vi "Traverse_to_Traverse_Collision.vi"(5 "Current Position":dbl[](array[numeric])=[0.0, 100.0, 40.0] format="%.2f", 7 "Traverse Name":string, 8 "Model  Roll        Pitch       Yaw (deg)":dbl[](array[numeric]) format="%#.2f", 9 "Work in Tunnel Coordinates":T1, 10 "Simulate/Run":T2=enum."Run VI", 11 "New Position":dbl[](array[numeric])=[0.0, 100.0, 40.0] format="%.2f") -> (1 "Error String":string)   [LabVIEW 2012]
uses:
  Controls/User_Specific_mode.ctl
  Controls/Tunnel_Coordinates.ctl
  Route mapping/Exclude_cluster.ctl
  Route mapping/Box_size.ctl
  Route mapping/Exclusion_type.ctl
  Controls/Global_mode.ctl
  Route mapping/Pict_Plot_Axis.ctl
  Route mapping/Axis.ctl
  Globals/Preference_global.vi
  Globals/Trav_pos_global.vi
panel:
  out "Plan View":picture
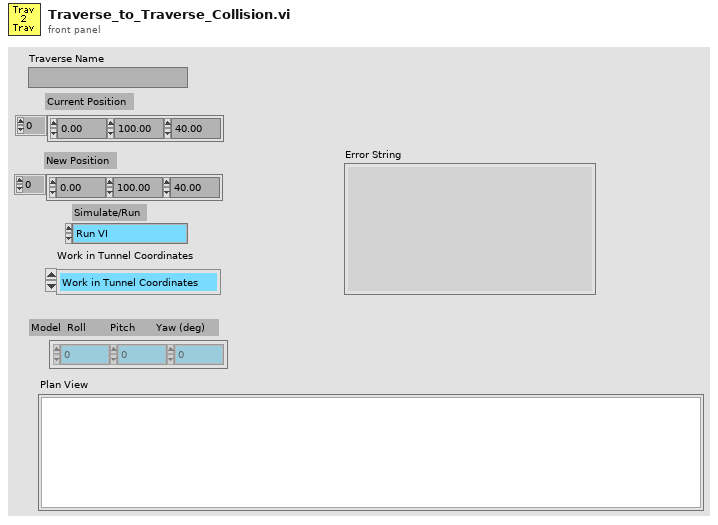
[diagram p1: front panel]
types:
  T1 = typedef "Tunnel_Coordinates.ctl" = enum16{"Work in Tunnel Coordinates", "Work in Model Coordinates"}
  T2 = typedef "User_Specific_mode.ctl" = enum16{"Check VI only", "Run VI"}
  T3 = typedef "Exclude_cluster.ctl" = cluster{"Sizes":T4, "Name":string, "Exclude Type":T5}
  T4 = typedef "Box_size.ctl" = cluster{"Max":dbl, "Min":dbl}[]
  T5 = typedef "Exclusion_type.ctl" = enum16{"Exclude completely", "Allow only vertical moves"}
  T6 = typedef "Global_mode.ctl" = enum16{"Read Global", "Load Global From File", "Write Global to File"}
  T7 = typedef "Pict_Plot_Axis.ctl" = cluster{"Width":T8, "Height":T8}
  T8 = typedef "Axis.ctl" = enum16{"X Axis", "X Axis -ve", "Y Axis", "Y Axis -ve", "Z Axis", "Z Axis -ve"}
  T9 = typedef "Update_scan_value.ctl" = cluster{"Channel Name":string, "New Value":dbl}
  T10 = enum16{"To Traverse Coordinates", "To User Coordinates"}
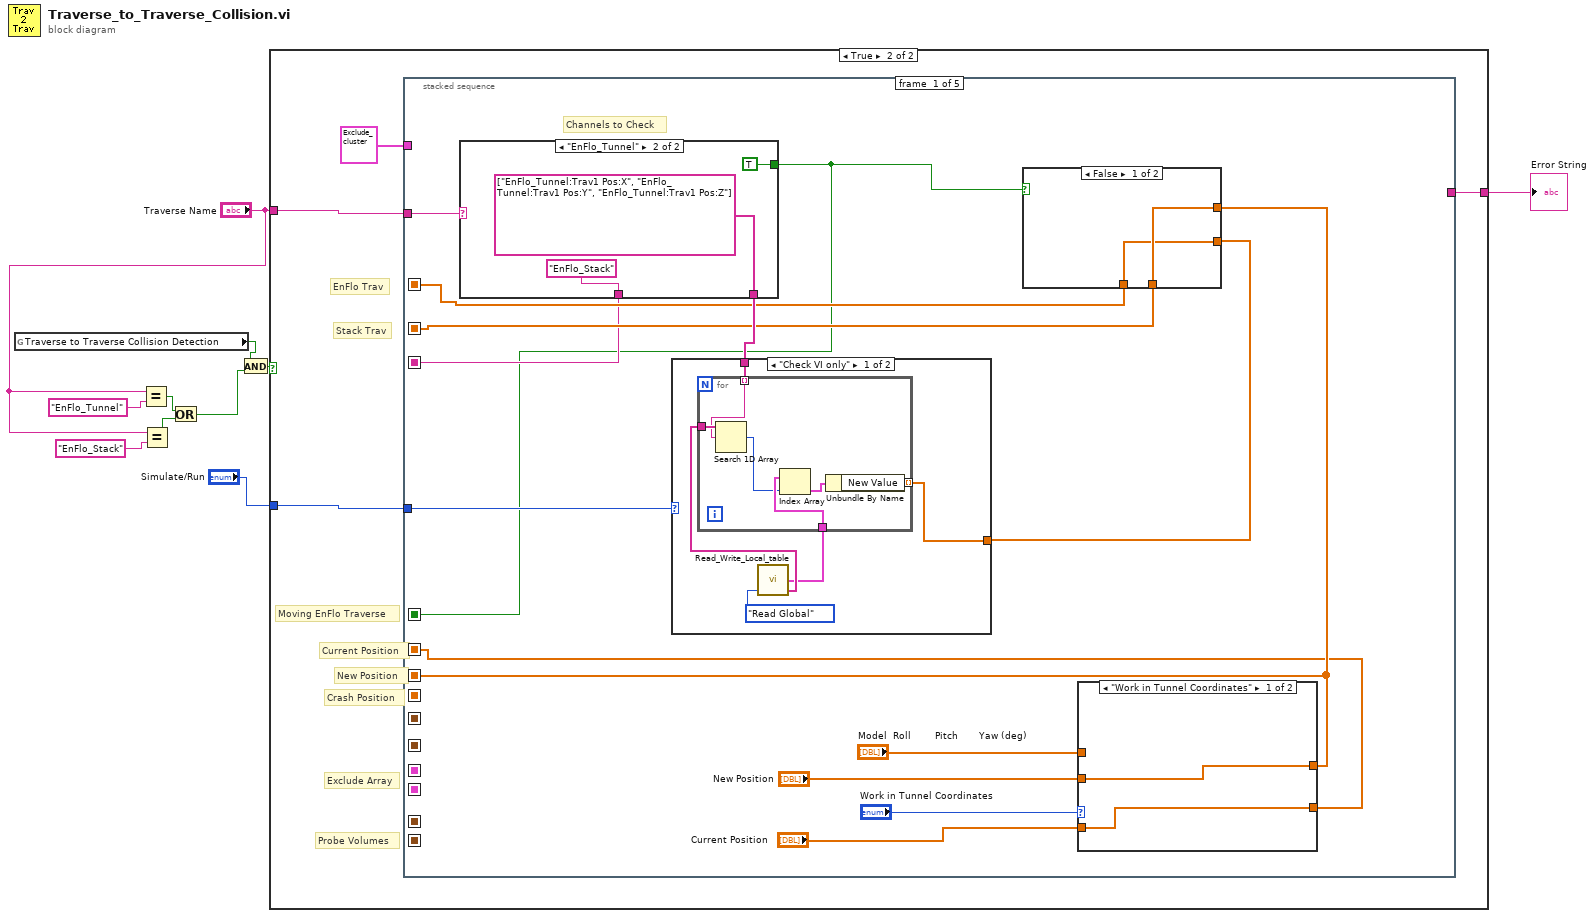
[diagram p0: block diagram]
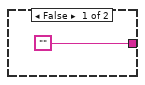
[diagram p2: hidden frame]
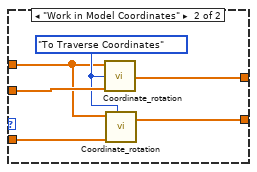
[diagram p4: hidden frame]
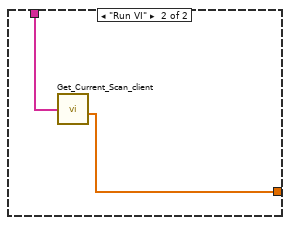
[diagram p5: hidden frame]
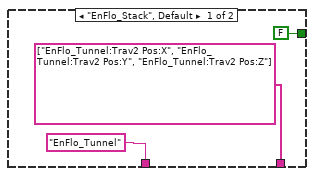
[diagram p6: hidden frame]
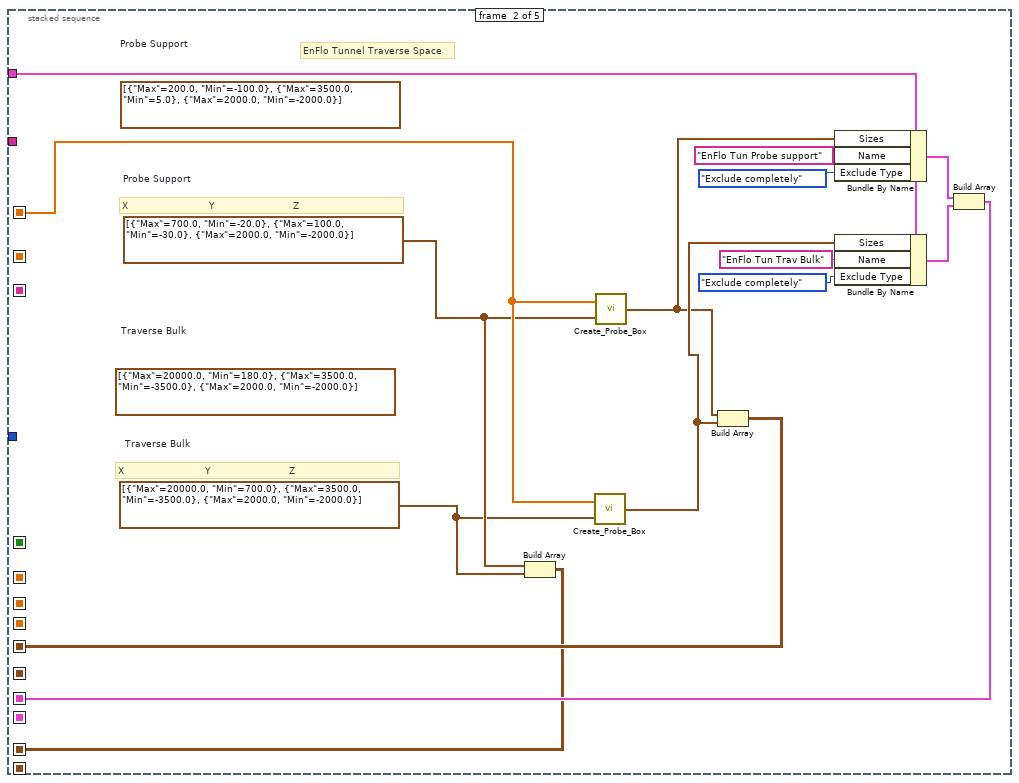
[diagram p7: hidden frame]
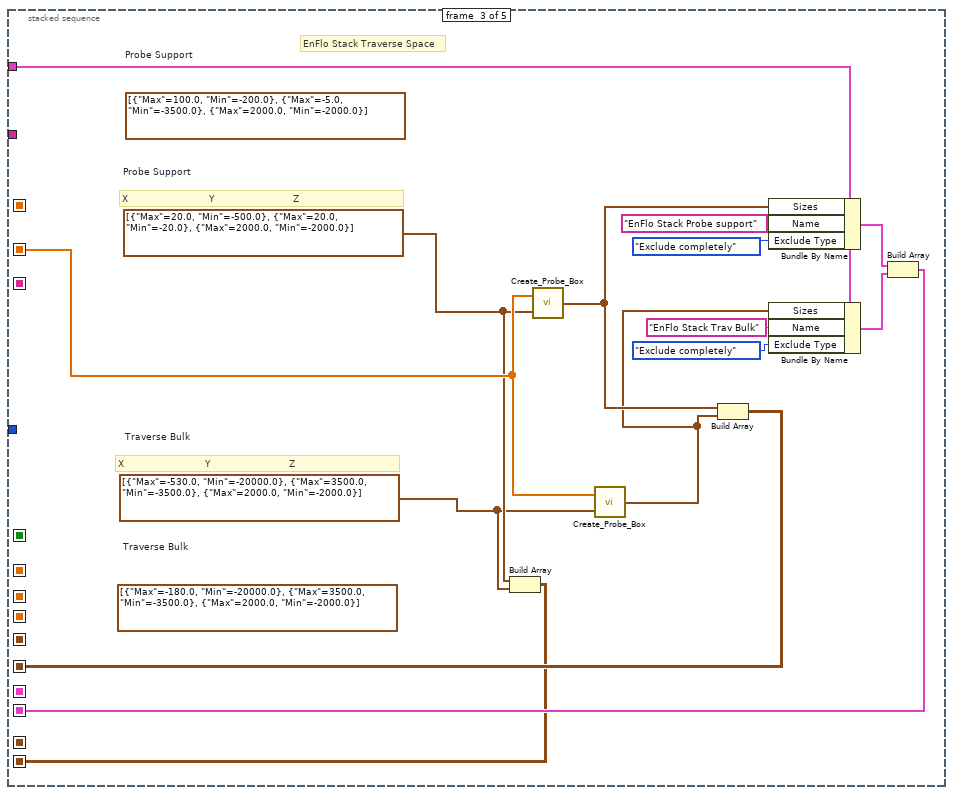
[diagram p8: hidden frame]
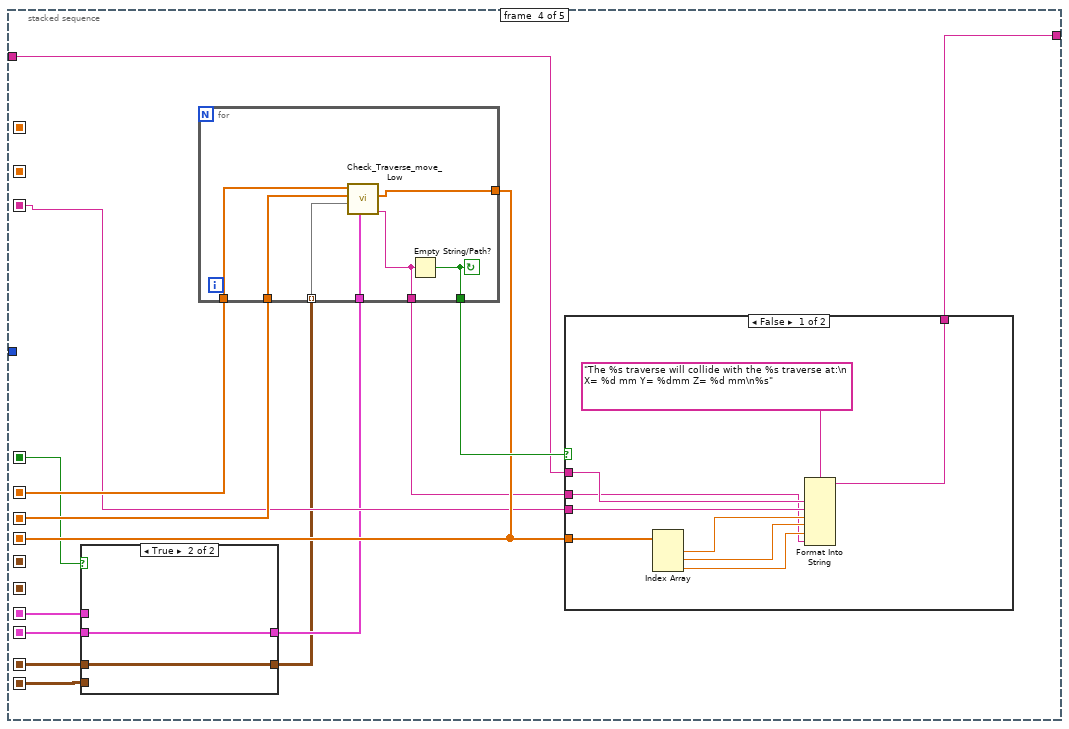
[diagram p9: hidden frame]
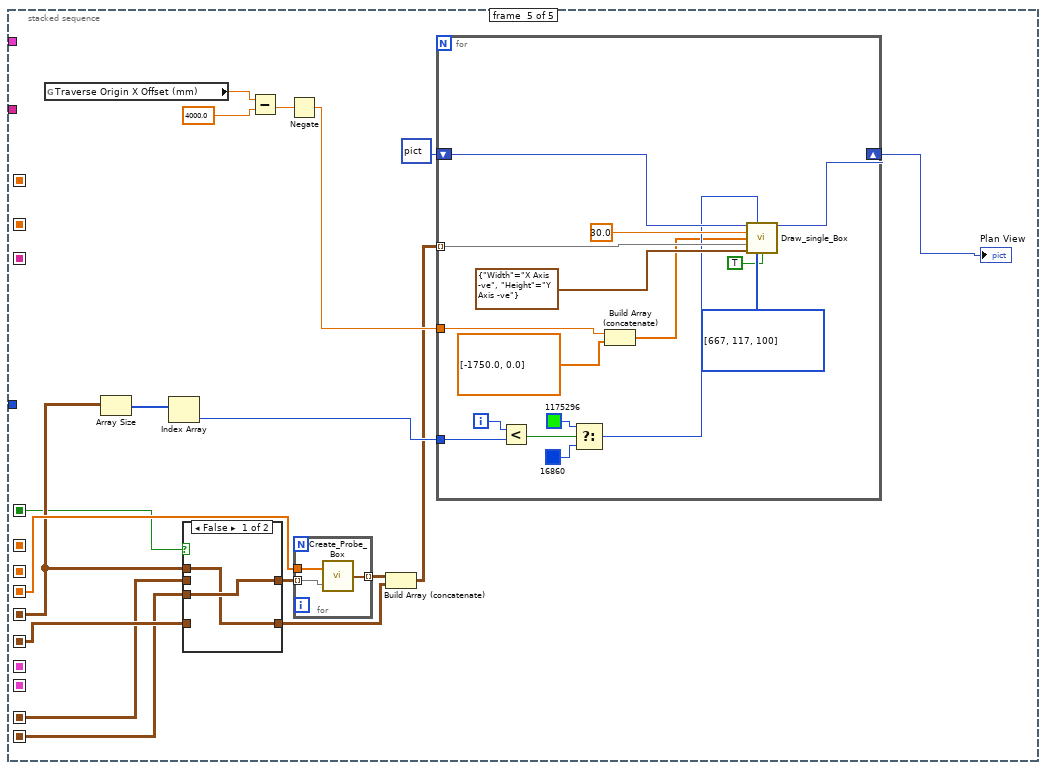
[diagram p12: hidden frame]
diagram:
  n1 = global read "Preference_global.vi" "Traverse to Traverse Collision Detection"() -> (w6:bool)
  n2 = Equal?(x="Traverse Name", y="EnFlo_Tunnel" ("Rig Setup")) -> (x = y?=w3:bool)
  n3 = Equal?(x="Traverse Name", y="EnFlo_Stack" ("Rig Setup")) -> (x = y?=w2:bool)
  n4 = Or(x=w3, y=w2) -> (x .or. y?=w1:bool)
  n5 = And(x=w6, y=w1) -> (x .and. y?=w7:bool)
  n6 = case shown="True" w7 {
    tunnel: "Traverse Name" -> [_ w15]
    tunnel: "Simulate/Run" -> [_ w14]
    tunnel: ["" w13] -> w8
    frame False {
    }
    frame True {
      # "Moving EnFlo Traverse"
      # "Exclude Array"
      # "Probe Volumes"
      # "Crash Position"
      # "Current Position"
      # "New Position"
      # "Stack Trav"
      # "EnFlo Trav"
      n7 = stacked-sequence {
        seq-local: [w23 _ _ _ _] -> [_ w75 _ _ _]
        seq-local: [w22 _ _ _ _] -> [_ _ w89 _ _]
        seq-local: [_ w74 _ _ _] -> [_ _ _ _ w128]
        seq-local: [_ _ w90 _ _] -> [_ _ _ _ w135]
        seq-local: [w20 _ _ _ _] -> [_ _ _ w100 _]
        seq-local: [w19 _ _ _ _] -> [_ _ _ w105 _]
        seq-local: [_ _ w80 _ _] -> [_ _ _ w97 _]
        seq-local: [_ w64 _ _ _] -> [_ _ _ w94 _]
        seq-local: [_ w61 _ _ _] -> [_ _ _ w95 w133]
        seq-local: [_ _ w76 _ _] -> [_ _ _ w93 w129]
        seq-local: [w17 _ _ _ _] -> [_ _ _ w104 _]
        seq-local: [_ _ _ w102 _] -> [_ _ _ _ w130]
        seq-local: [w16 _ _ _ _] -> [_ _ _ w91 w127]
        tunnel: w15 -> [w27 _ _ w101 _]
        tunnel: w14 -> [w29 _ _ _ _]
        tunnel: [_ _ _ w99 _] -> w13
        tunnel: T3 {"Sizes"=[{"Max"=15000.0, "Min"=0.0}, {"Max"=1000.0, "Min"=-1000.0}, {"Max"=300.0, "Min"=0.0}], "Name"="Roughness Elements", "Exclude Type"=enum."Allow only vertical moves"} ("Cluster") -> [_ w65 w79 _ _]
        frame #0 {
          # "Channels to Check"
          n8 = case shown="\"EnFlo_Tunnel\"" w27 {
            tunnel: [string[] ["EnFlo_Tunnel:Trav2 Pos:X", "EnFlo_Tunnel:Trav2 Pos:Y", "EnFlo_Tunnel:Trav2 Pos:Z"] string[] ["EnFlo_Tunnel:Trav1 Pos:X", "EnFlo_Tunnel:Trav1 Pos:Y", "EnFlo_Tunnel:Trav1 Pos:Z"]] -> w28
            tunnel: [FALSE TRUE] -> w16
            tunnel: ["EnFlo_Tunnel" "EnFlo_Stack"] -> w20
            frame "EnFlo_Stack", Default {
            }
            frame "EnFlo_Tunnel" {
            }
          }
          n9 = case shown="\"Check VI only\"" w29 {
            tunnel: [w42 w53] -> w21
            tunnel: w28 -> [w44 w54]
            frame "Check VI only" {
              n10 = call "Read_Write_Local_table.vi"("Mode"=Global_mode."Read Global") -> ("Ch Names"=w45:string[], "Ch Values Out"=w43:T9[])  [unwired: 2 in, 1 out]
              n11 = for {
                tunnel: w45 -> [w52]
                tunnel: w44 -> [w51] mode=indexing
                tunnel: w43 -> [w50]
                tunnel: [w47] -> w42 mode=indexing
                n12 = Search 1D Array(1D array=w52, element=w51) -> (index of element=w49:i32)  [unwired: 1 out]
                n13 = Index Array(array=w50, index=w49) -> (element=w48:T9)
                n14 = Unbundle By Name(w48) -> ("New Value"=w47:dbl)
              }
            }
            frame "Run VI" {
              n15 = call "Get_Current_Scan_client.vi"("ADAM Ch Names"=w54) -> ("Numerical Values"=w53:dbl[])  [unwired: 3 out]
            }
          }
          n16 = case shown="\"Work in Tunnel Coordinates\"" "Work in Tunnel Coordinates" {
            tunnel: "Model  Roll        Pitch       Yaw (deg)" -> [_ w38]
            tunnel: "New Position" -> [w35 w41]
            tunnel: [w35 w40] -> w19
            tunnel: "Current Position" -> [w34 w37]
            tunnel: [w34 w36] -> w17
            frame "Work in Tunnel Coordinates" {
            }
            frame "Work in Model Coordinates" {
              w39 = T10."To Traverse Coordinates" ("Mode")
              n17 = call "Coordinate_rotation.vi"("Model       Roll      Pitch       Yaw (deg)"=w38, "Input Position"=w41, "Mode"=w39) -> ("Output Position"=w40:dbl[])  [unwired: 2 in, 1 out]
              n18 = call "Coordinate_rotation.vi"("Model       Roll      Pitch       Yaw (deg)"=w38, "Input Position"=w37, "Mode"=w39) -> ("Output Position"=w36:dbl[])  [unwired: 2 in, 1 out]
            }
          }
          n19 = case shown="False" w16 {
            tunnel: [w30 w33] -> w23
            tunnel: w19 -> [w31 w33]
            tunnel: [w31 w32] -> w22
            tunnel: w21 -> [w30 w32]
            frame False {
            }
            frame True {
            }
          }
        }
        frame #1 {
          (unwired) T4 [{"Max"=20000.0, "Min"=180.0}, {"Max"=3500.0, "Min"=-3500.0}, {"Max"=2000.0, "Min"=-2000.0}]  # Traverse Bulk
          (unwired) T4 [{"Max"=200.0, "Min"=-100.0}, {"Max"=3500.0, "Min"=5.0}, {"Max"=2000.0, "Min"=-2000.0}]  # Probe Support
          w62 = T4 [{"Max"=20000.0, "Min"=700.0}, {"Max"=3500.0, "Min"=-3500.0}, {"Max"=2000.0, "Min"=-2000.0}]  # Traverse Bulk
          w63 = T4 [{"Max"=700.0, "Min"=-20.0}, {"Max"=100.0, "Min"=-30.0}, {"Max"=2000.0, "Min"=-2000.0}]  # Probe Support
          # "X                           Y                          Z"
          # "EnFlo Tunnel Traverse Space"
          # "X                           Y                          Z"
          n20 = Build Array(w63, w62) -> (w61:cluster{"Max":dbl, "Min":dbl}[][])
          n21 = call "Create_Probe_Box.vi"("Probe Volume"=w62, "Probe Position"=w75) -> ("Current Probe Volume"=w67:cluster{"Max":dbl, "Min":dbl}[])
          n22 = call "Create_Probe_Box.vi"("Probe Volume"=w63, "Probe Position"=w75) -> ("Current Probe Volume"=w66:cluster{"Max":dbl, "Min":dbl}[])
          n23 = Build Array(w66, w67) -> (w74:cluster{"Max":dbl, "Min":dbl}[][])
          n24 = Bundle By Name(cluster=w65, "Sizes"=w66, "Name"="EnFlo Tun Probe support", "Exclude Type"=Exclusion_type."Exclude completely") -> (w68:T3)
          n25 = Bundle By Name(cluster=w65, "Sizes"=w67, "Name"="EnFlo Tun Trav Bulk", "Exclude Type"=Exclusion_type."Exclude completely") -> (w69:T3)
          n26 = Build Array(w68, w69) -> (w64:T3[])
        }
        frame #2 {
          (unwired) T4 [{"Max"=-180.0, "Min"=-20000.0}, {"Max"=3500.0, "Min"=-3500.0}, {"Max"=2000.0, "Min"=-2000.0}]  # Traverse Bulk
          (unwired) T4 [{"Max"=100.0, "Min"=-200.0}, {"Max"=-5.0, "Min"=-3500.0}, {"Max"=2000.0, "Min"=-2000.0}]  # Probe Support
          w77 = T4 [{"Max"=-530.0, "Min"=-20000.0}, {"Max"=3500.0, "Min"=-3500.0}, {"Max"=2000.0, "Min"=-2000.0}]  # Traverse Bulk
          w78 = T4 [{"Max"=20.0, "Min"=-500.0}, {"Max"=20.0, "Min"=-20.0}, {"Max"=2000.0, "Min"=-2000.0}]  # Probe Support
          # "X                           Y                          Z"
          # "EnFlo Stack Traverse Space"
          # "X                           Y                          Z"
          n27 = Build Array(w78, w77) -> (w76:cluster{"Max":dbl, "Min":dbl}[][])
          n28 = call "Create_Probe_Box.vi"("Probe Volume"=w78, "Probe Position"=w89) -> ("Current Probe Volume"=w88:cluster{"Max":dbl, "Min":dbl}[])
          n29 = call "Create_Probe_Box.vi"("Probe Volume"=w77, "Probe Position"=w89) -> ("Current Probe Volume"=w84:cluster{"Max":dbl, "Min":dbl}[])
          n30 = Build Array(w88, w84) -> (w90:cluster{"Max":dbl, "Min":dbl}[][])
          n31 = Bundle By Name(cluster=w79, "Sizes"=w88, "Name"="EnFlo Stack Probe support", "Exclude Type"=Exclusion_type."Exclude completely") -> (w81:T3)
          n32 = Bundle By Name(cluster=w79, "Sizes"=w84, "Name"="EnFlo Stack Trav Bulk", "Exclude Type"=Exclusion_type."Exclude completely") -> (w82:T3)
          n33 = Build Array(w81, w82) -> (w80:T3[])
        }
        frame #3 {
          n34 = case shown="True" w91 {
            tunnel: [w107 w109] -> w98
            tunnel: w97 -> [_ w109]
            tunnel: [w106 w108] -> w96
            tunnel: w95 -> [_ w108]
            tunnel: w94 -> [w107 _]
            tunnel: w93 -> [w106 _]
            frame False {
            }
            frame True {
            }
          }
          n35 = for {
            tunnel: w105 -> [w126]
            tunnel: w104 -> [w125]
            tunnel: w98 -> [w124]
            tunnel: w96 -> [w123] mode=indexing
            tunnel: [w122] -> w102
            tunnel: [w121] -> w103
            tunnel: [w120] -> w92
            stop <- w121 continue-if-true
            n36 = call "Check_Traverse_move_Low.vi"("Exclude Array"=w124, "Probe Volume"=w123, "New Position"=w126, "Current position"=w125) -> ("Error Comments"=w120:string, "Position At Crash"=w122:dbl[])  [unwired: 4 in]
            n37 = Empty String/Path?(string/path=w120) -> (empty?=w121:bool)
          }
          n38 = case shown="False" w103 {
            tunnel: [w116 w119] -> w99
            tunnel: w92 -> [w110 w119]
            tunnel: w101 -> [w111 _]
            tunnel: w100 -> [w117 _]
            tunnel: w102 -> [w115 _]
            frame False {
              n39 = Index Array(array=w115) -> (element #1=w112:dbl, element #2=w114:dbl, element #3=w113:dbl)  [unwired: 3 in]
              n40 = Format Into String(format string="The %s traverse will collide with the %s traverse at:\n X= %d mm Y= %dmm Z= %d mm\n%s" ("Format String"), w111, w117, w112, w114, w113, w110) -> (resulting string=w116:string)  [unwired: 2 in, 1 out]
            }
            frame True {
            }
          }
        }
        frame #4 {
          n41 = global read "Trav_pos_global.vi" "Traverse Origin X Offset (mm)"() -> (w139:dbl)
          n42 = Array Size(array=w128) -> (size(s)=w142:i32[])
          n43 = Index Array(array=w142) -> (element=w141:i32)  [unwired: 1 in]
          n44 = case shown="False" w127 {
            tunnel: [w148 w151] -> w136
            tunnel: w135 -> [_ w151]
            tunnel: w133 -> [_ w150]
            tunnel: [w149 w150] -> w132
            tunnel: w129 -> [w149 _]
            tunnel: w128 -> [w148 _]
            frame False {
            }
            frame True {
            }
          }
          n45 = Subtract(x=w139, y=4000.0 ("x")) -> (x-y=w137:dbl)
          n46 = Negate(x=w137) -> (-x=w140:dbl)
          n47 = for {
            tunnel: w132 -> [w147] mode=indexing
            tunnel: [w146] -> w131 mode=indexing
            tunnel: w130 -> [w145]
            n48 = call "Create_Probe_Box.vi"("Probe Volume"=w147, "Probe Position"=w145) -> ("Current Probe Volume"=w146:cluster{"Max":dbl, "Min":dbl}[])
          }
          n49 = Build Array (concatenate)(w131, w136) -> (w134:cluster{"Max":dbl, "Min":dbl}[][])
          n50 = for {
            shift-right: [w164] -> w143
            shift-left: picture data[5B] ("Picture in") -> [w165]
            tunnel: w134 -> [w163] mode=indexing
            tunnel: w141 -> [w159]
            tunnel: w140 -> [w153]
            i -> [w160]
            n51 = Less?(x=w160, y=w159) -> (x < y?=w158:bool)
            n52 = Select(t=u32 1175296 ("color(black)"), s=w158, f=u32 16860 ("color(black)")) -> (s? t:f=w155:u32)
            n53 = Build Array (concatenate)(w153, dbl[] [-1750.0, 0.0] ("Min Values")) -> (w152:dbl[])
            n54 = call "Draw_single_Box.vi"("Picture in"=w165, "color(black)"=w155, "mm Per Pixel"=30.0, "Min Values"=w152, "Box Coordinates"=w163, "View"=T7 {"Width"=enum."X Axis -ve", "Height"=enum."Y Axis -ve"}, "Pixels per Axis"=i16[] [667, 117, 100], "fill?(F)"=TRUE) -> ("Picture out"=w164:picture)  [unwired: 7 out]
          }
          "Plan View" <- w143
        }
      }
    }
  }
  "Error String" <- w8
